vi "ALTS-2015 Flush TCP Buffer.vi"(8 "error in (no error)":errorcluster, 11 "TCP Connection in":refnum<k5>) -> (0 "error out":errorcluster, 3 "TCP Connection out":refnum<k5>)   [LabVIEW 2013]
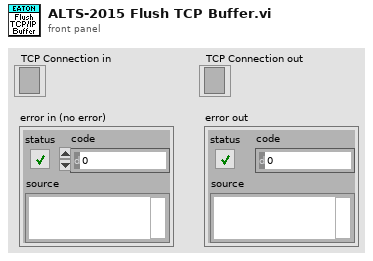
[diagram p1: front panel]
types:
  T1 = enum16{"Standard", "Buffered", "CRLF", "Immediate"}
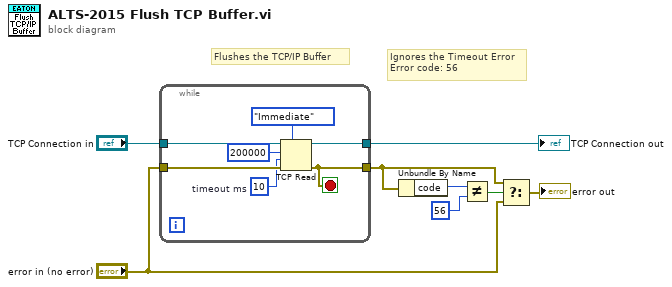
[diagram p0: block diagram]
diagram:
  # "Ignores the Timeout Error\nError code: 56"
  # "Flushes the TCP/IP Buffer"
  n1 = while {
    tunnel: "error in (no error)" -> [w15]
    tunnel: [w10] -> w6
    tunnel: "TCP Connection in" -> [w14]
    tunnel: [w13] -> w2
    stop <- w10 stop-if-true
    w11 = 10  # timeout ms
    n2 = TCP Read(connection ID=w14, bytes to read=200000, error in (no error)=w15, 7:T1."Immediate" ("mode (standard)"), 9:w11) -> (connection ID out=w13:refnum<k5>, error out=w10:errorcluster)  [unwired: 1 out]
  }
  "TCP Connection out" <- w2
  n3 = Unbundle By Name(w6) -> ("code"=w3:i32)
  n4 = Not Equal?(x=w3, y=56) -> (x != y?=w5:bool)
  n5 = Select(t=w6, s=w5, f="error in (no error)") -> (s? t:f=→"error out":errorcluster)
